vi "FTW-CodeGen-Image.vi"(0 "State In":T1 {"Cache"."TotalCodeGens" format="CodeGens:   %04d"; "Cache"."TotalAdaptToInputs" format="AdaptTerms: %04d"; "Cache"."FinishedCodegen" format="%_3psec"; "Cache"."ElapsedTilCodegen" format="%_3psec"; "Cache"."AdaptToInputsBegin" format="%.3fmsec\n%<%D:%H:%M:%S%3u>t"}, 5 "XRef":refnum<vi>) -> (4 "Image":picture)   [LabVIEW 2015, in "FTW-Actor-Ask.xnode"]
uses:
  FTW-Actor-Ask.xnode
  FTW-CodeGen-State.ctl
  FTW-CodeGen-XNodeCommonState.ctl
  FTW-CodeGen-XNodeAdaptiveTerminal.ctl
  FTW-CodeGen-XNodeAdaptiveTerminal-Controller.ctl
  src/reflection/FTW-Reflection-Types.ctl
  FTW-CodeGen-XNodeAdaptiveTerminalWiringBehavior.ctl
panel:
  # "Inputs"
  # "Outputs"
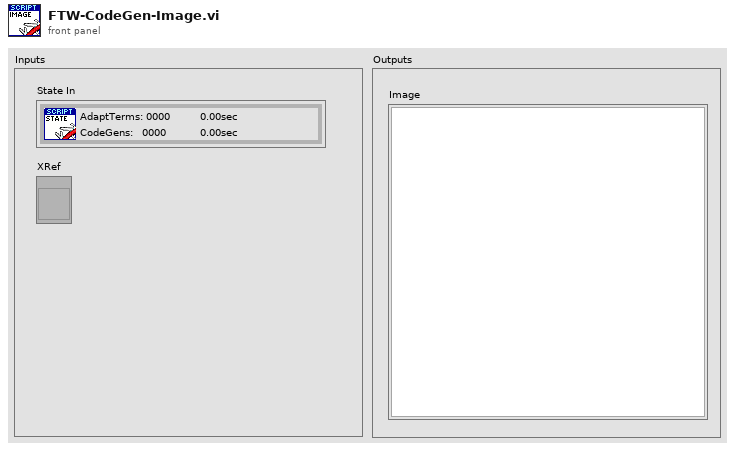
[diagram p1: front panel]
types:
  T1 = typedef "FTW-Actor-Ask.xnode/FTW-CodeGen-State.ctl" = cluster{"Cache":T2}
  T2 = typedef "FTW-CodeGen-XNodeCommonState.ctl" = cluster{"Terms":cluster{"Name":string, "Id":string, "Type":variant, "Bounds":cluster{"Left":i32, "Top":i32, "Right":i32, "Bottom":i32}, "Input?":bool, "Required?":bool, "Recommended?":bool, "Adaptive?":bool, "Hidden?":bool, "Direction":enum32{"Auto", "Up", "Down", "Left", "Right", "Center"}, "Break Wire?":bool, "English Name":string}[], "AdaptiveTerms":T3[], "AdaptiveTerminalsOK":bool, "ForceCodeRegeneration?":bool, "LastGeneration":timestamp, "CodeGenError":errorcluster, "AdaptToInputsBegin":dbl, "ElapsedTilCodegen":dbl, "FinishedCodegen":dbl, "TotalAdaptToInputs":i32, "TotalCodeGens":i32}
  T3 = typedef "FTW-CodeGen-XNodeAdaptiveTerminal.ctl" = cluster{"Config":T4, "ID":string, "ParentIndex":i32, "Wired?":bool, "WiredTypeAllowed?":bool, "LastValidWireName":string, "LastValidWireType":T5, "Followers":i32[]}
  T4 = typedef "FTW-CodeGen-XNodeAdaptiveTerminal-Controller.ctl" = cluster{"AllowedTypes":T5[], "UnconstrainedTypeBehavior":T6, "DefaultType":variant}
  T5 = typedef "FTW-Reflection-Types.ctl" = enum16{"Unknown", "Void", "Array", "Cluster", "LVObject", "Boolean", "I8", "I16", "I32", "I64", "U8", "U16", "U32", "U64", "SGL", "DBL", "EXT", "CSG", "CDB", "CXT", "FXP", "EnumU8", "EnumU16", "EnumU32", "EnumU64", "SGLwithUnit", "DBLwithUnit", "EXTwithUnit", "CSGwithUnit", "CDBwithUnit", "CXTwithUnit", "String", "Path", "Picture", "Tag", "LVVariant", "Timestamp", "WaveformI8", "WaveformI16", "WaveformI32", "WaveformI64", "WaveformU8", "WaveformU16", "WaveformU32", "WaveformU64", "WaveformSGL", "WaveformDBL", "WaveformEXT", "WaveformCSG", "WaveformCDB", "WaveformCXT", "WaveformDigital", "WaveformUnknownType", "DigitalData", "DynamicData", "ExternalData", "FileByteStream", "TDMStream", "dotNET", "ActiveX", "VIServerReference", "VIReference", "ApplicationInstance", "Menu", "ConnectionDataSocket", "ConnectionVISA", "ConnectionBluetooth", "ConnectionIrDA", "ConnectionTCP", "ConnectionUDP", "ConnectionHTTPClient", "ConnectionFTP", "Occurrence", "Notifier", "Queue", "Rendezvous", "Semaphore", "RTFIFO", "EventPublisher", "EventRegistration", "EventCallback", "DataValueReference", "GenericClass", "GenericClassTag", "GenericClassDeepCopy", "GenericClassFlattened", "GenericClassTagFlattened", "GenericReferenceType", "WindowsRegistry", "OverloadedDatalogRef", "ReferenceUnknownType", "ByteArray", "ConPaneInterface", "FTWObject"}
  T6 = typedef "FTW-CodeGen-XNodeAdaptiveTerminalWiringBehavior.ctl" = enum16{"UseDefaultType", "StickyToLastValidType"}
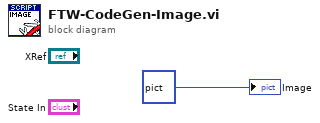
[diagram p0: block diagram]
diagram:
  "Image" <- picture bytes[3102]
